vi "LLchecker2.vi"() -> ()   [LabVIEW 2013]
uses:
  <vilib>/nisyscfg/Find Systems.vi
  <vilib>/nisyscfg/Close (System).vi
  <vilib>/nisyscfg/nisyscfg.lvlib
  <resource>/objmgr/nisysapi.rc
panel:
  in  "subsets":string[](array[string])=["rtats", "rtperf", "rtint"] caption="Target name subsets to monitor"
  out "Log":string
  out "Email Error":errorcluster caption="error out"
  in  "Email Recipients (CSV)":string="brian.frantz@ni.com, chris.carson@ni.com"
  out "Monitored Systems":T1(array[cluster])
  in  "# of \nOfflines to Notify":i32[](array[numeric])=[5, 600]
  out "Last update":timestamp
  out "Refresh Error":errorcluster
  out "New Target Error":errorcluster
  in  "New Target Scan Interval (min):":u32=60
  in  "Refresh Interval (min):":i32=5
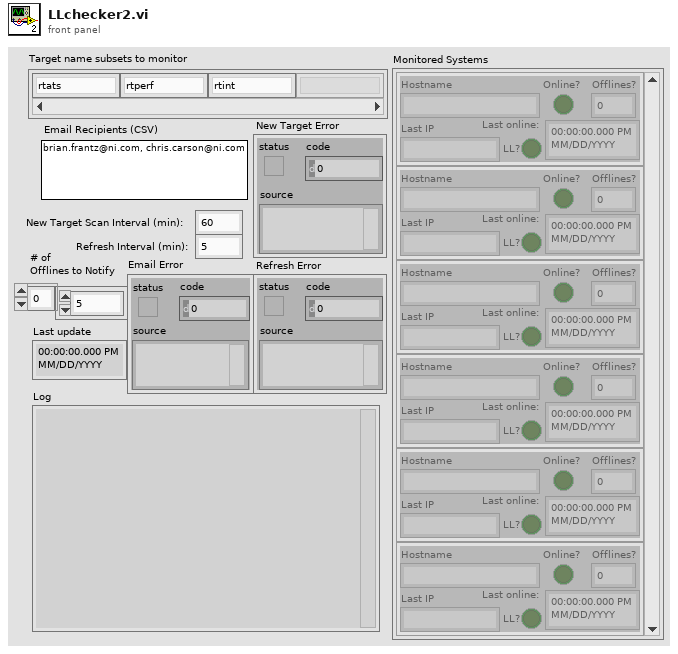
[diagram p1: front panel]
types:
  T1 = cluster{"Hostname":string, "Online?":bool, "Last online:":timestamp, "Offlines?":i32, "Last IP":string, "LL?":bool}[]
  T2 = cluster{"Hostname":string, "Online?":bool, "Last online:":timestamp, "Offlines?":i32, "Last IP":string, "LL?":bool}
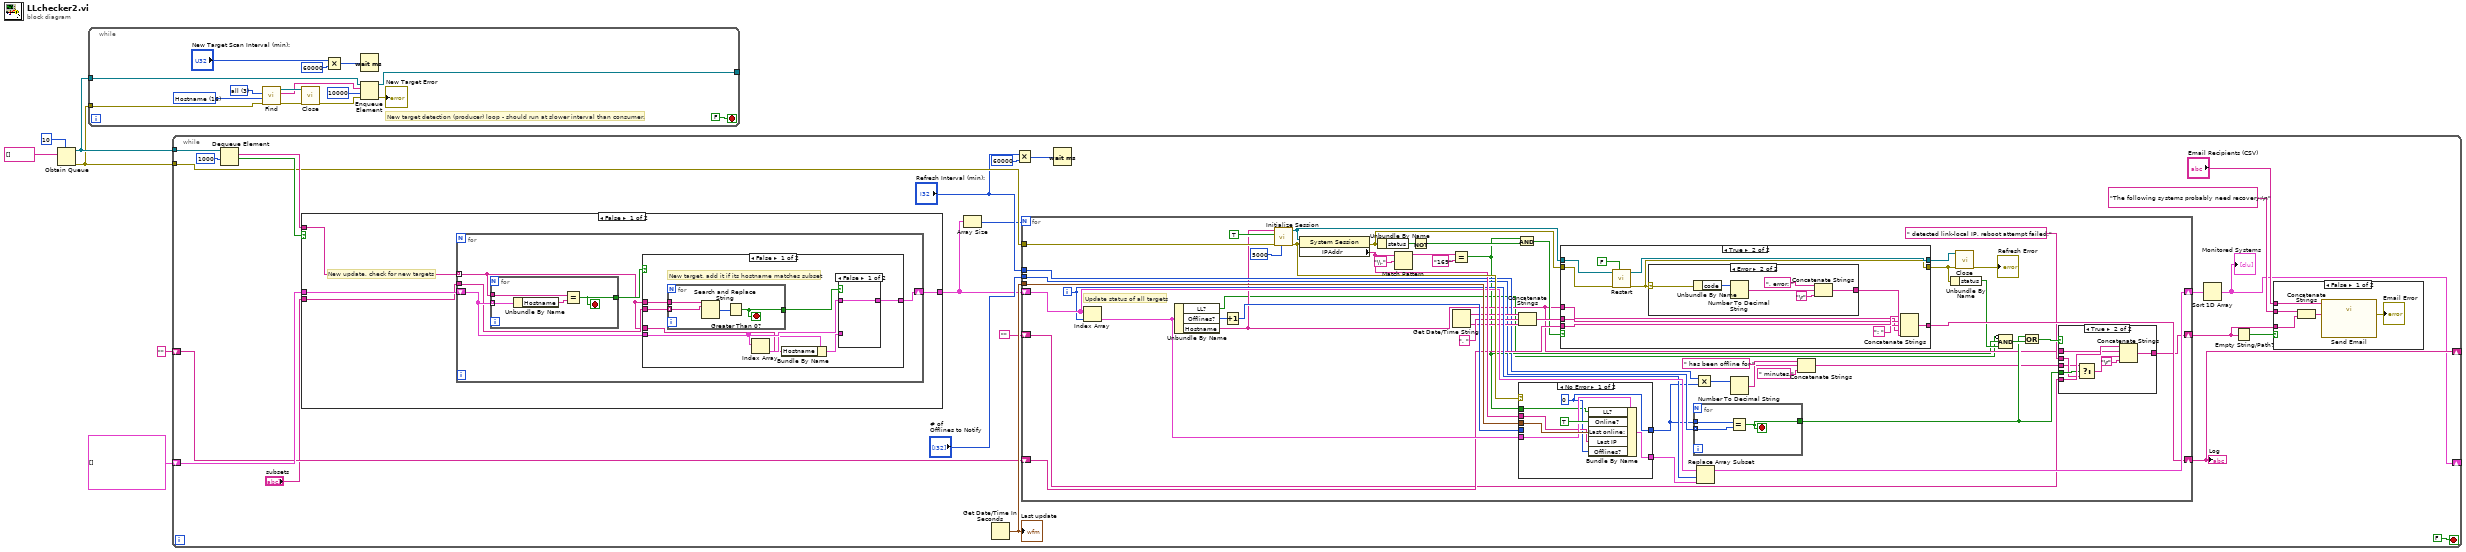
[diagram p0: block diagram]
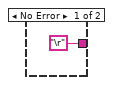
[diagram p5: hidden frame]
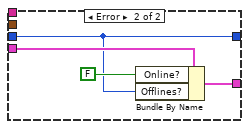
[diagram p6: hidden frame]
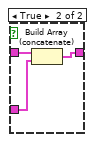
[diagram p7: hidden frame]
diagram:
  n1 = Obtain Queue(max queue size (-1, unlimited)=10, element data type=string[] [] ("detected systems")) -> (queue out=w4:refnum<queue>, error out=w3:errorcluster)  [unwired: 3 in, 1 out]
  n2 = while {
    tunnel: w4 -> [w12]
    tunnel: w3 -> [w13]
    tunnel: [w8] -> _
    stop <- FALSE stop-if-true
    w18 = u32 16 items=["Hostname"=16, "Hostname (IP)"=18, "Hostname (MAC)"=19, "IP"=32, "IP (Hostname)"=33, "IP (MAC)"=35, "MAC"=48, "MAC (Hostname)"=49, "MAC (IP)"=50] ("output (hostname and IP)")
    w17 = u32 3 items=["none"=0, "only if online"=1, "all"=3] ("include cached results (all)")
    # "New target detection (producer) loop - should run at slower interval than consumer."
    n3 = call-poly <vilib>:"Find.vi"("error in (no error)"=w13, "output (hostname and IP)"=w18, "include cached results (all)"=w17) -> ("error out"=w16:errorcluster, "detected systems"=w10:string[], "session out"=w15:refnum<k21>)  [unwired: 6 in]
    n4 = call-poly <vilib>:"Close.vi"("error in (no error)"=w16, "session in"=w15) -> ("error out"=w14:errorcluster)  [unwired: 9 in]
    n5 = Multiply(x="New Target Scan Interval (min):", y=u32 60000) -> (x*y=w21:u32)
    n6 = Wait (ms)(milliseconds to wait=w21) -> ()  [unwired: 1 out]
    n7 = Enqueue Element(queue=w12, element=w10, timeout in ms (-1)=10000, error in (no error)=w14) -> (queue out=w8:refnum<queue>, error out=→"New Target Error":errorcluster)  [unwired: 1 out]
  }
  n8 = while {
    tunnel: w4 -> [w43]
    tunnel: w3 -> [w37]
    shift-right: [w22] -> _
    shift-left: T1 [] ("Monitored Systems") -> [w40]
    shift-right: [w33] -> _
    shift-left: "" ("Log") -> [w34]
    stop <- FALSE stop-if-true
    n9 = Dequeue Element(queue=w43, timeout in ms (-1)=1000) -> (element=w39:string[], timed out?=w41:bool)  [unwired: 1 in, 2 out]
    n10 = case shown="False" w41 {
      tunnel: w40 -> [w145 w173]
      tunnel: w39 -> [w146 _]
      tunnel: [w144 w173] -> w25
      tunnel: "subsets" -> [w143 _]
      frame False {
        # "New update, check for new targets"
        n11 = for {
          tunnel: w146 -> [w147] mode=indexing
          shift-right: [w149] -> w144
          shift-left: w145 -> [w150]
          tunnel: w143 -> [w148]
          n12 = for {
            tunnel: w150 -> [w171] mode=indexing
            tunnel: w147 -> [w172]
            tunnel: [w169] -> w151
            stop <- w169 stop-if-true
            n13 = Unbundle By Name(w171) -> ("Hostname"=w170:string)
            n14 = Equal?(x=w172, y=w170) -> (x = y?=w169:bool)
          }
          n15 = case shown="False" w151 {
            tunnel: w150 -> [w159 w168]
            tunnel: w147 -> [w156 _]
            tunnel: [w155 w168] -> w149
            tunnel: w148 -> [w154 _]
            tunnel: w147 -> [w153 _]
            frame False {
              # "New target, add it if its hostname matches subset"
              n16 = for {
                tunnel: w154 -> [w165] mode=indexing
                tunnel: [w166] -> w152
                tunnel: w153 -> [w164]
                stop <- w166 stop-if-true
                n17 = Search and Replace String(input string=w164, search string=w165) -> (number of replacements=w167:i32)  [unwired: 6 in, 3 out]
                n18 = Greater Than 0?(x=w167) -> (x > 0?=w166:bool)
              }
              n19 = Index Array(array=w159) -> (element=w158:T2)  [unwired: 1 in]
              n20 = Bundle By Name(cluster=w158, "Hostname"=w156) -> (w157:T2)
              n21 = case shown="False" w152 {
                tunnel: w159 -> [w160 w163]
                tunnel: w157 -> [_ w162]
                tunnel: [w160 w161] -> w155
                frame False {
                }
                frame True {
                  n22 = Build Array (concatenate)(w163, w162) -> (w161:T1)
                }
              }
            }
            frame True {
              # "Existing, do \nnothing."
            }
          }
        }
      }
      frame True {
      }
    }
    n23 = Array Size(array=w25) -> (size(s)=w24:i32)
    n24 = Get Date/Time In Seconds() -> (seconds since 1Jan1904=w36:timestamp)
    "Last update" <- w36
    n25 = Multiply(x="Refresh Interval (min):", y=60000) -> (x*y=w45:i32)
    n26 = for {
      N: w24 -> [_]
      tunnel: w37 -> [w96]
      tunnel: w36 -> [w91]
      shift-right: [w83] -> w35
      shift-left: w25 -> [w86]
      shift-right: [w79] -> w33
      shift-left: w34 -> [w80]
      shift-right: [w57] -> w27
      shift-left: "" ("Log") -> [w72]
      tunnel: "# of \nOfflines to Notify" -> [w71]
      tunnel: "Refresh Interval (min):" -> [w64]
      i -> [w85]
      # "Update status of all targets"
      n27 = Index Array(array=w86, index=w85) -> (element=w87:T2)
      n28 = Unbundle By Name(w87) -> ("LL?"=w51:bool, "Offlines?"=w89:i32, "Hostname"=w63:string)
      n29 = Increment(x=w89) -> (x+1=w88:i32)
      n30 = call <vilib>:"Initialize Session.vi"("connect timeout in ms (4s)"=u32 5000, "error in (no error)"=w96, "force property refresh (T)"=TRUE, "target (localhost)"=w63) -> ("error out"=w92:errorcluster, "session out"=w55:refnum<k21>)  [unwired: 6 in]
      n31 = property class="System Session"(reference=w55, error in=w92) -> (error out=w81:errorcluster, "IPAddr"=w90:string)  [unwired: 1 out]
      n32 = Unbundle By Name(w81) -> ("status"=w73:bool)
      n33 = Match Pattern(string=w90, regular expression="\\.") -> (before substring=w93:string)  [unwired: 1 in, 3 out]
      n34 = Not(x=w73) -> (.not. x?=w82:bool)
      n35 = Equal?(x=w93, y="169") -> (x = y?=w56:bool)
      n36 = Get Date/Time String() -> (date string=w78:string, time string=w75:string)  [unwired: 3 in]
      n37 = And(x=w56, y=w82) -> (x .and. y?=w74:bool)
      n38 = Concatenate Strings(w78, ", " ("string"), w75) -> (w76:string)
      n39 = case shown="No Error" w92 {
        tunnel: w87 -> [w136 w142]
        tunnel: w91 -> [w137 _]
        tunnel: w90 -> [w135 _]
        tunnel: [w134 w141] -> w84
        tunnel: w88 -> [_ w139]
        tunnel: [w133 w139] -> w65
        tunnel: w56 -> [w132 _]
        frame No Error {
          w133 = 0 ("Offlines?")
          n40 = Bundle By Name(cluster=w136, "LL?"=w132, "Online?"=TRUE, "Last online:"=w137, "Last IP"=w135, "Offlines?"=w133) -> (w134:T2)
        }
        frame Error {
          n41 = Bundle By Name(cluster=w142, "Online?"=FALSE, "Offlines?"=w139) -> (w141:T2)
        }
      }
      n42 = case shown="True" w74 {
        tunnel: w55 -> [w112 w123]
        tunnel: w81 -> [w111 w122]
        tunnel: w80 -> [w113 w120]
        tunnel: [w113 w119] -> w79
        tunnel: w76 -> [_ w118]
        tunnel: w63 -> [_ w116]
        tunnel: [w111 w114] -> w53
        tunnel: [w112 w115] -> w54
        frame False {
        }
        frame True {
          n43 = call <vilib>:"Restart.vi"("wait until complete (T)"=FALSE, "error in (no error)"=w122, "session in"=w123) -> ("error out"=w114:errorcluster, "session out"=w115:refnum<k21>)  [unwired: 6 in, 1 out]
          n44 = case shown="Error" w114 {
            selector: w114 -> [_ w131]
            tunnel: ["\r" w126] -> w121
            frame No Error {
            }
            frame Error {
              n45 = Unbundle By Name(w131) -> ("code"=w130:i32)
              n46 = Number To Decimal String(number=w130) -> (decimal integer string=w129:string)  [unwired: 1 in]
              n47 = Concatenate Strings(", error: " ("string"), w129, "\r") -> (w126:string)
            }
          }
          n48 = Concatenate Strings(w120, w118, ": " ("string"), w116, w121) -> (w119:string)
        }
      }
      n49 = for {
        tunnel: w71 -> [w101] mode=indexing
        tunnel: w65 -> [w100]
        tunnel: [w99] -> w67
        stop <- w99 stop-if-true
        n50 = Equal?(x=w100, y=w101) -> (x = y?=w99:bool)
      }
      n51 = Multiply(x=w64, y=w65) -> (x*y=w62:i32)
      n52 = Replace Array Subset(array=w86, new element=w84, index=w85) -> (w83:T1)
      n53 = Number To Decimal String(number=w62) -> (decimal integer string=w60:string)  [unwired: 1 in]
      n54 = Concatenate Strings(" has been offline for " ("Hostname"), w60, " minutes." ("string")) -> (w58:string)
      n55 = Unbundle By Name(w53) -> ("status"=w70:bool)
      n56 = call-poly <vilib>:"Close.vi"("error in (no error)"=w53, "session in"=w54) -> ("error out"=→"Refresh Error":errorcluster)  [unwired: 9 in]
      n57 = Compound Arithmetic op=AND(invert w51, w56, w70) -> (w69:bool)
      n58 = Or(x=w67, y=w69) -> (x .or. y?=w68:bool)
      n59 = case shown="True" w68 {
        tunnel: w67 -> [_ w107]
        tunnel: w72 -> [w102 w109]
        tunnel: w63 -> [_ w108]
        tunnel: " detected link-local IP, reboot attempt failed." ("Hostname") -> [_ w106]
        tunnel: w58 -> [_ w104]
        tunnel: [w102 w105] -> w57
        frame False {
        }
        frame True {
          n60 = Select(t=w104, s=w107, f=w106) -> (s? t:f=w103:string)
          n61 = Concatenate Strings(w109, w108, w103, "\r") -> (w105:string)
        }
      }
    }
    "Log" <- w33
    n62 = Wait (ms)(milliseconds to wait=w45) -> ()  [unwired: 1 out]
    n63 = Sort 1D Array(array=w35) -> (sorted array=w22:T1)
    "Monitored Systems" <- w22
    n64 = Empty String/Path?(string/path=w27) -> (empty?=w29:bool)
    n65 = case shown="False" w29 {
      tunnel: "Email Recipients (CSV)" -> [w50 _]
      tunnel: w27 -> [w49 _]
      tunnel: "The following systems probably need recovery:\n" ("string") -> [w46 _]
      frame False {
        n66 = Concatenate Strings(w46, w49) -> (w47:string)
        n67 = call "Send Email"("Message"=w47, "Recipients"=w50) -> ("error out"=→"Email Error":errorcluster)  [unwired: 9 in]
      }
      frame True {
        # "No need to notify."
      }
    }
  }
